vi "Destroy.vi"(8 "error in (no error)":errorcluster, 11 "Engine in":refnum<class "Engine.lvclass">) -> (0 "error out":errorcluster)   [LabVIEW 2019, in "RT_Game.lvlib" / "Engine.lvclass"]
uses:
  Engine.lvclass
  Engine.lvclass/Engine.ctl
  <vilib>/FPGAPlugInAG/myRIO-1900/niLvFpga_Close_myRIO-1900.vi
  Globals.vi
  Game/Game.lvclass
  <vilib>/rvi/interface/nirviCloseFPGA/nirviCloseFPGA.xnode
  FPGA_Interface.ctl
  FPGA Bitfiles/myriogameconsole_FPGATarget_Main_ntsPRcBZGxk.lvbitx
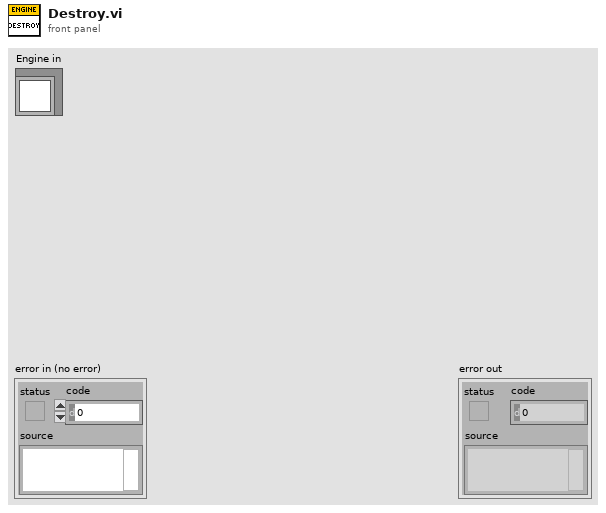
[diagram p1: front panel]
types:
  T1 = typedef "FPGA_Interface.ctl" = refnum<k20>
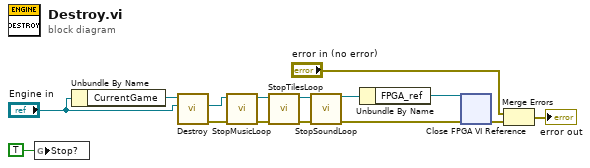
[diagram p0: block diagram]
diagram:
  n1 = global write "Globals.vi" "Stop?"(TRUE ("Stop?")) -> ()
  n2 = Unbundle By Name("Engine in") -> ("CurrentGame"=w10:refnum<class "Game.lvclass">)
  n3 = call-dynamic "Destroy.vi"("RT_Game.lvlib:Engine.lvclass"="Engine in", "Game in"=w10) -> ("error out"=w12:errorcluster, "RT_Game.lvlib:Engine.lvclass 2"=w8:refnum<class "Engine.lvclass">)  [unwired: 8 in]
  n4 = call "StopMusicLoop.vi"("error in (no error)"=w12, "Engine in"=w8) -> ("error out"=w9:errorcluster, "Engine out"=w6:refnum<class "Engine.lvclass">)  [unwired: 8 in]
  n5 = call "StopTilesLoop.vi"("error in (no error)"=w9, "Engine in"=w6) -> ("error out"=w7:errorcluster, "Engine out"=w4:refnum<class "Engine.lvclass">)  [unwired: 8 in]
  n6 = call "StopSoundLoop.vi"("error in (no error)"=w7, "Engine in"=w4) -> ("error out"=w5:errorcluster, "Engine out"=w2:refnum<class "Engine.lvclass">)  [unwired: 8 in]
  n7 = Unbundle By Name(w2) -> ("FPGA_ref"=w1:T1)
  n8 = xnode "Close FPGA VI Reference"("FPGA VI Reference In"=w1, "error in"=w5) -> ("error out"=w11:errorcluster)
  n9 = Merge Errors("error in (no error)", w11) -> (→"error out":errorcluster)
